vi "NI_controller_Feedback.VI"(1 "Initialize":bool=TRUE, 6 "Z Position (mm)":dbl format="%.3f", 8 "Motion System":T1=enum."No Motion Card", 9 "Y Position (mm)":dbl format="%.3f", 10 "X Position (mm)":dbl format="%.3f", 11 "Motion ID":T2=1 min=1 max=32 step=1) -> (0 "error out":errorcluster)   [LabVIEW 2022 SP3]
uses:
  <vilib>/Motion/FlexMotion/CustomControls/CustomControls.llb/AxisOrVectorSpace To Configure.flx
  <vilib>/Motion/FlexMotion/FunctionsVIs/StartStopMotion.llb/Start Motion (8 axes).flx
  <vilib>/Motion/FlexMotion/FunctionsVIs/StartStopMotion.llb/Stop Motion (8 axes).flx
  -MotionRoutines/MotionGlobals.vi
  <vilib>/Motion/FlexMotion/FunctionsVIs/Trajectory.llb/Load Acceleration/Deceleration.flx
  -NI_MotionRoutines/MotionSys.ctl
panel:
  in  "Slave Axis":u16(ring)=2 items=["Axis 1"=1, "Axis 2"=2, "Axis 3"=3, "Axis 4"=4]
  in  "Master Axis":u16(ring)=1 items=["Axis 1"=1, "Axis 2"=2, "Axis 3"=3, "Axis 4"=4]
  in  "Enable Gearing":bool
  out "Angle":dbl=45.000038009906035
  in  "Ratio Denom":u16=1 min=1 max=32767
  in  "Ratio Num":i16 min=0
  in  "Center 4":bool
  in  "Acceleration":i32=100000
  in  "Velocity":i32=20000
  in  "Position":dbl format="%.3f"
  in  "FineMi4":bool
  in  "FinePl4":bool
  in  "Rst4":bool
  in  "Ax4Plus":bool
  in  "Ax4Minus":bool
  in  "FineMi3":bool
  in  "FinePl3":bool
  in  "Rst3":bool
  in  "Ax3Plus":bool
  in  "Ax3Minus":bool
  in  "FineMi2":bool
  in  "FinePl2":bool
  in  "Rst2":bool
  in  "Ax2Plus":bool
  in  "Ax2Minus":bool
  in  "stop":bool
  in  "FineMi1":bool
  in  "FinePl1":bool
  in  "Rst1":bool
  in  "Ax1Plus":bool
  in  "Ax1Minus":bool
  # "Units are in mm. \"Rst\" zeros the position. Blue circles move 1 cm for linear."
  # "Be very careful with this mode it is not fully programmed"
  # "X Axis"
  # "Y Axis"
  # "Centers linear actuator"
  # "Z Axis"
  # "LinInd/Rotational Axis"
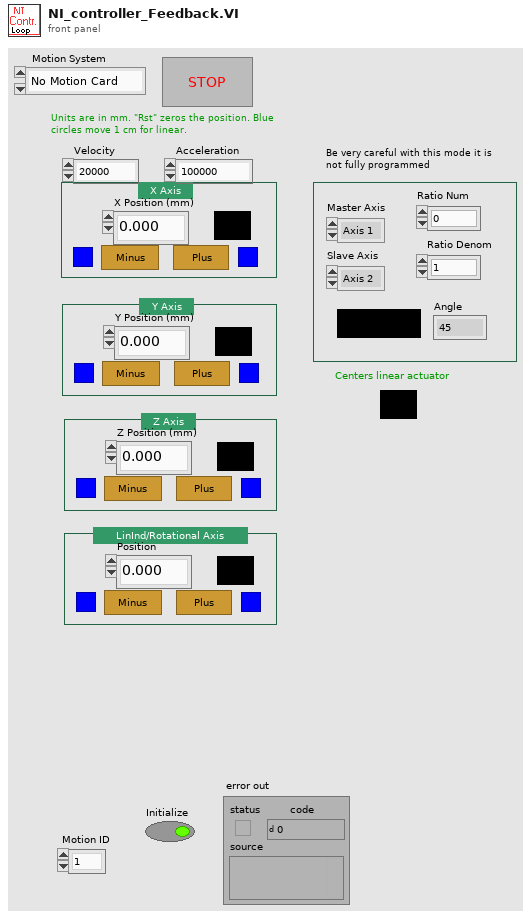
[diagram p1: front panel]
types:
  T1 = typedef "MotionSys.ctl" = enum16{"MM3000", "NI 735x", "Newport ESP", "No Motion Card", "Galil"}
  T2 = typedef "Board Id" = u8
  T3 = typedef "Bd Id Out" = u8
  T4 = typedef "location.ctl" = enum16{"Automatic", "WCM Main", "Hawaii", "Columbia MM3000", "Columbia  NI System", "NYU", "RRI 2", "UHI Allen", "CUMC RT", "Chiba", "Stony Brook", "WCM Microscopy", "WCM Aeoretch", "WCM Optics Lab", "WCM Main 2Axis", "WCM Rotation", "WCM SAM SMAC", "SERI GP"}
  T5 = typedef "AxisOrVectorSpace To Configure.flx" = u16
  T6 = enum16{"Absolute Position", "Relative Position", "Velocity", "Relative to Cap Pos", "Modulus Position", "Absolute Contouring", "Relative Contouring"}
  T7 = typedef "Resource Out (Enum).flx" = u16
  T8 = typedef "Axis Status (8 axes).flx" = cluster{"1":bool, "2":bool, "3":bool, "4":bool, "5":bool, "6":bool, "7":bool, "8":bool}
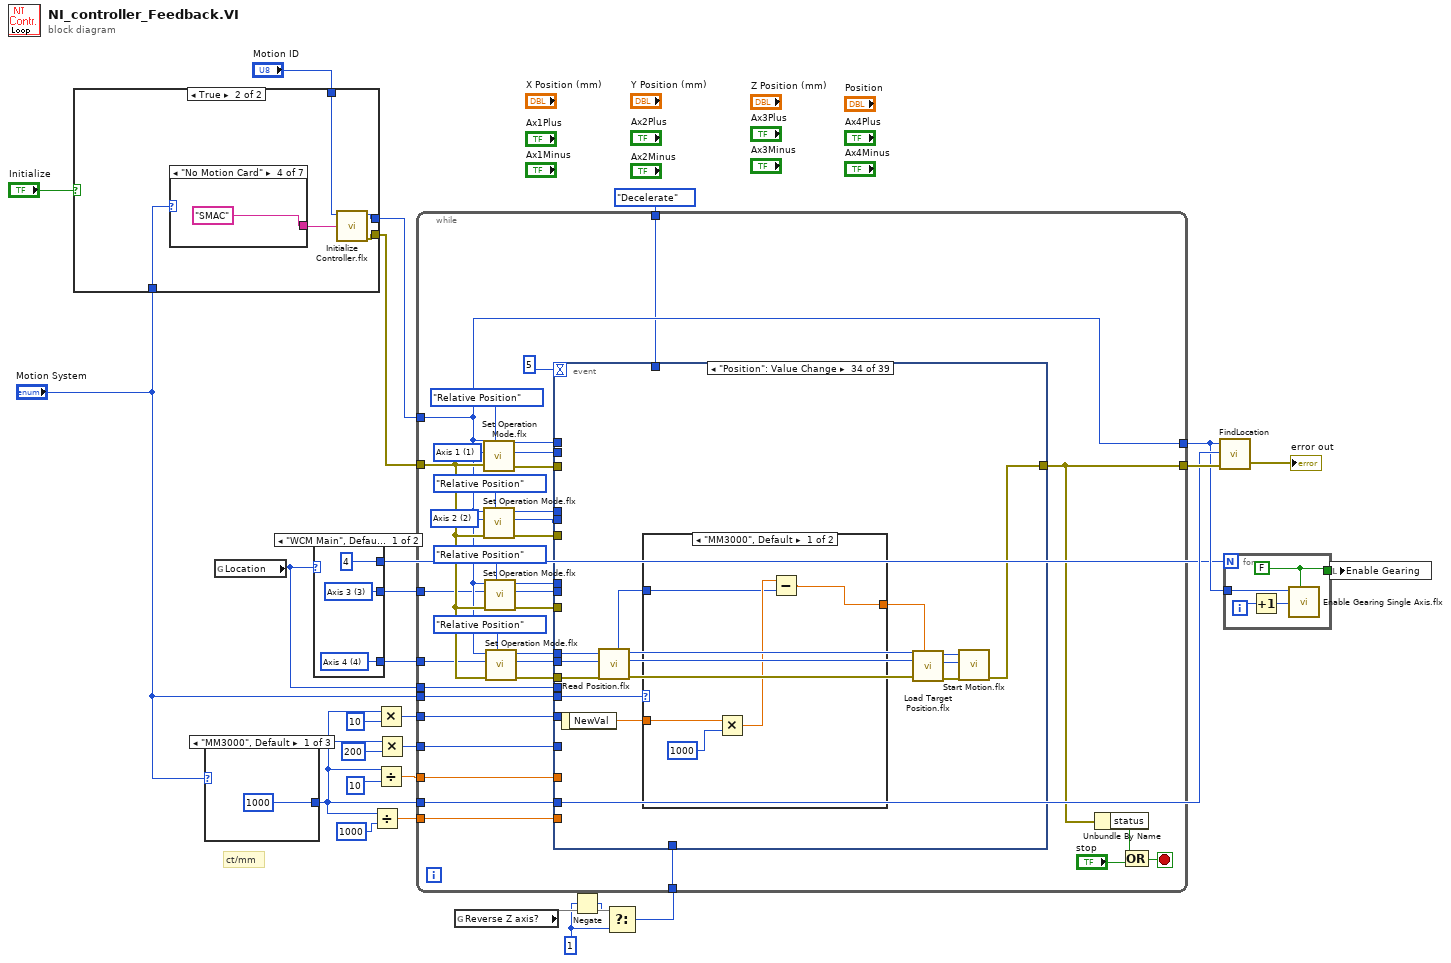
[diagram p0: block diagram]
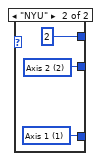
[diagram p2: hidden frame]
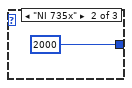
[diagram p3: hidden frame]
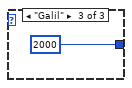
[diagram p4: hidden frame]
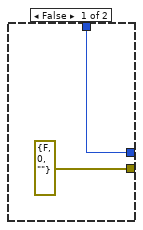
[diagram p5: hidden frame]
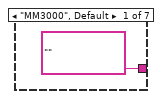
[diagram p6: hidden frame]
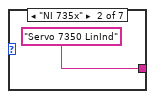
[diagram p7: hidden frame]
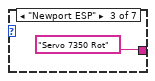
[diagram p8: hidden frame]
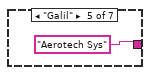
[diagram p9: hidden frame]
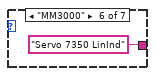
[diagram p10: hidden frame]
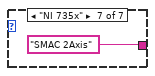
[diagram p11: hidden frame]
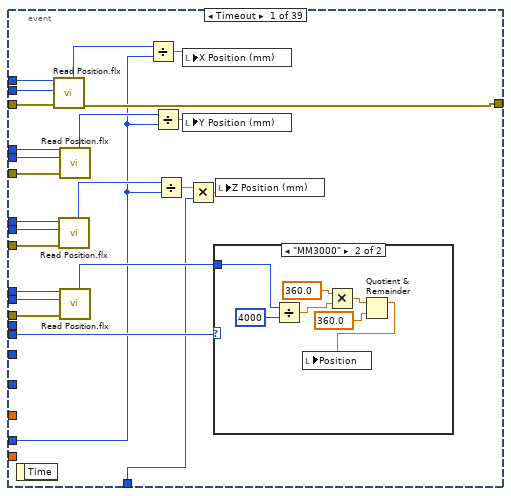
[diagram p12: hidden frame]
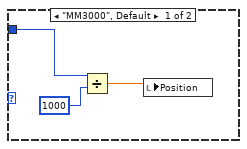
[diagram p13: hidden frame]
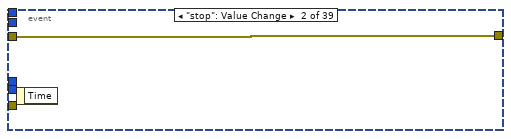
[diagram p14: hidden frame]
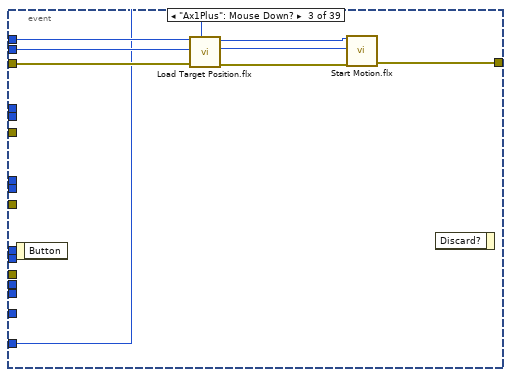
[diagram p15: hidden frame]
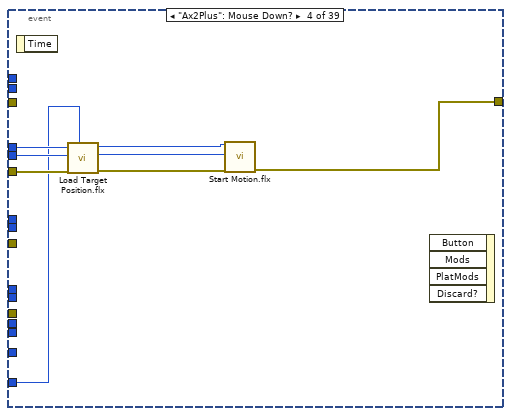
[diagram p16: hidden frame]
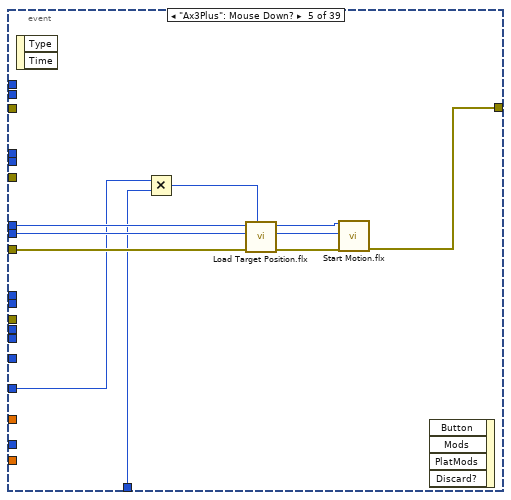
[diagram p17: hidden frame]
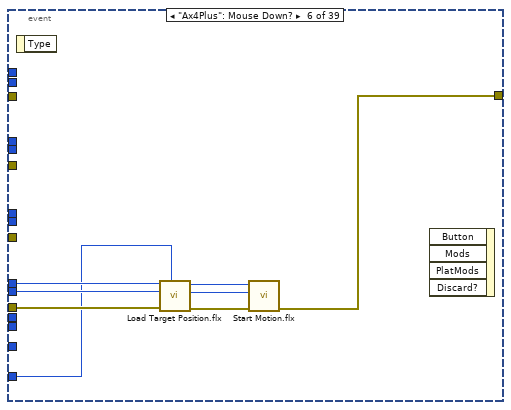
[diagram p18: hidden frame]
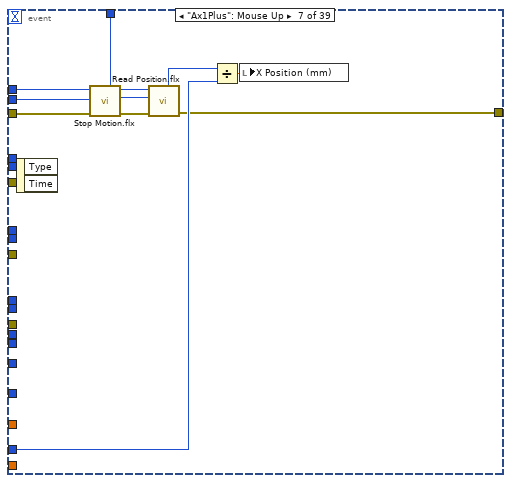
[diagram p19: hidden frame]
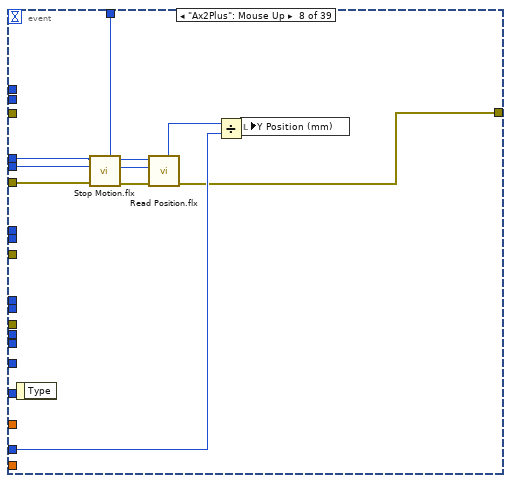
[diagram p20: hidden frame]
diagram:
  w12 = 1
  # "ct/mm"
  n1 = case shown="True" "Initialize" {
    tunnel: [w29 w34] -> w27
    tunnel: [errorcluster {"status"=FALSE, "code"=0, "source"=""} ("error out") w33] -> w26
    tunnel: "Motion ID" -> [w29 w31]
    tunnel: "Motion System" -> [_ w30]
    frame False {
    }
    frame True {
      n2 = case shown="\"No Motion Card\"" w30 {
        tunnel: ["" "Servo 7350 LinInd" "Servo 7350 Rot" "SMAC" "Aerotech Sys" "Servo 7350 LinInd" "SMAC 2Axis"] -> w32
        frame "MM3000", Default {
        }
        frame "NI 735x" {
        }
        frame "Newport ESP" {
        }
        frame "No Motion Card" {
        }
        frame "Galil" {
        }
        frame "MM3000" {
        }
        frame "NI 735x" {
        }
      }
      n3 = call <vilib>:"Initialize Controller.flx"("Settings Name"=w32, "Board ID"=w31) -> ("error out"=w33:errorcluster, "Bd ID Out"=w34:T3)  [unwired: 1 in, 5 out]
    }
  }
  n4 = case shown="\"MM3000\", Default" "Motion System" {
    tunnel: [1000 ("y") 2000 ("y") 2000 ("y")] -> w7
    frame "MM3000", Default {
    }
    frame "NI 735x" {
    }
    frame "Galil" {
    }
  }
  n5 = global read "MotionGlobals.vi" "Location"() -> (w1:T4)
  n6 = case shown="\"WCM Main\", Default" w1 {
    tunnel: [w47 w49] -> w4
    tunnel: [w46 w50] -> w3
    tunnel: [4 2] -> w2
    frame "WCM Main", Default {
      w47 = T5 4 items=["Axis 1"=1, "Axis 2"=2, "Axis 3"=3, "Axis 4"=4, "Axis 5"=5, "Axis 6"=6, "Vector Space 1"=17, "Vector Space 2"=18, "Vector Space 3"=19] ("Axis or Vector Space")
      w46 = T5 3 items=["Axis 1"=1, "Axis 2"=2, "Axis 3"=3, "Axis 4"=4, "Axis 5"=5, "Axis 6"=6, "Vector Space 1"=17, "Vector Space 2"=18, "Vector Space 3"=19] ("Axis or Vector Space")
    }
    frame "NYU" {
      w49 = T5 1 items=["Axis 1"=1, "Axis 2"=2, "Axis 3"=3, "Axis 4"=4, "Axis 5"=5, "Axis 6"=6, "Vector Space 1"=17, "Vector Space 2"=18, "Vector Space 3"=19] ("Axis or Vector Space")
      w50 = T5 2 items=["Axis 1"=1, "Axis 2"=2, "Axis 3"=3, "Axis 4"=4, "Axis 5"=5, "Axis 6"=6, "Vector Space 1"=17, "Vector Space 2"=18, "Vector Space 3"=19] ("Axis or Vector Space")
    }
  }
  n7 = Divide(x=w7, y=1000) -> (x/y=w10:dbl)
  n8 = Multiply(x=w7, y=10) -> (x*y=w14:i32)
  n9 = Divide(x=w7, y=10) -> (x/y=w17:dbl)
  n10 = Multiply(x=w7, y=200) -> (x*y=w13:i32)
  n11 = global read "MotionGlobals.vi" "Reverse Z axis?"() -> (w22)
  n12 = Negate(x=w12) -> (-x=w21:i32)
  n13 = Select(t=w21, s=w22, f=w12) -> (s? t:f=w20:i32)
  n14 = while {
    tunnel: [w58] -> w23
    tunnel: w26 -> [w74]
    tunnel: w27 -> [w66]
    tunnel: [w66] -> w6
    tunnel: w20 -> [w62]
    tunnel: w17 -> [w61]
    tunnel: w7 -> [w60]
    tunnel: "Motion System" -> [w59]
    tunnel: w14 -> [w57]
    tunnel: w13 -> [w56]
    tunnel: w10 -> [w55]
    tunnel: enum16{"Decelerate", "Halt", "Kill"}."Decelerate" ("Stop Type (Decel)") -> [w54]
    tunnel: w4 -> [w53]
    tunnel: w3 -> [w52]
    tunnel: w1 -> [w51]
    stop <- w85 stop-if-true
    w63 = T5 2 items=["Axis 1"=1, "Axis 2"=2, "Axis 3"=3, "Axis 4"=4, "Axis 5"=5, "Axis 6"=6, "Vector Space 1"=17, "Vector Space 2"=18, "Vector Space 3"=19] ("Axis or Vector Space")
    w79 = T5 1 items=["Axis 1"=1, "Axis 2"=2, "Axis 3"=3, "Axis 4"=4, "Axis 5"=5, "Axis 6"=6, "Vector Space 1"=17, "Vector Space 2"=18, "Vector Space 3"=19] ("Axis or Vector Space")
    n15 = call <vilib>:"Set Operation Mode.flx"("Position Mode (Absolute)"=T6."Relative Position", "error in (no error)"=w74, "Axis or Vector Space"=w79, "Board ID"=w66) -> ("error out"=w81:errorcluster, "Resource Output"=w78:T7, "Bd ID Out"=w82:T3)  [unwired: 2 out]
    n16 = call <vilib>:"Set Operation Mode.flx"("Position Mode (Absolute)"=T6."Relative Position", "error in (no error)"=w74, "Axis or Vector Space"=w63, "Board ID"=w66) -> ("error out"=w73:errorcluster, "Resource Output"=w65:T7, "Bd ID Out"=w64:T3)  [unwired: 2 out]
    n17 = call <vilib>:"Set Operation Mode.flx"("Position Mode (Absolute)"=T6."Relative Position", "error in (no error)"=w74, "Axis or Vector Space"=w52, "Board ID"=w66) -> ("error out"=w70:errorcluster, "Resource Output"=w71:T7, "Bd ID Out"=w72:T3)  [unwired: 2 out]
    n18 = call <vilib>:"Set Operation Mode.flx"("Position Mode (Absolute)"=T6."Relative Position", "error in (no error)"=w74, "Axis or Vector Space"=w53, "Board ID"=w66) -> ("error out"=w67:errorcluster, "Resource Output"=w68:T7, "Bd ID Out"=w69:T3)  [unwired: 2 out]
    n19 = event shown="[33] \"Position\": Value Change" {
      selector: _ -> [_ _ _ _ _ _ _ _ _ _ _ _ _ _ _ _ _ _ _ _ _ _ _ _ _ _ _ _ _ _ _ _ _ _ _ _ _ _ _]
      dyn-events: _ -> [_ _ _ _ _ _ _ _ _ _ _ _ _ _ _ _ _ _ _ _ _ _ _ _ _ _ _ _ _ _ _ _ _ _ _ _ _ _ _]
      timeout: 5 -> [_ _ _ _ _ _ _ _ _ _ _ _ _ _ _ _ _ _ _ _ _ _ _ _ _ _ _ _ _ _ _ _ _ _ _ _ _ _ _]
      tunnel: w82 -> [w110 _ w129 _ _ _ w166 _ _ _ w227 _ _ _ w266 _ _ _ w324 _ _ _ w344 _ _ _ w400 _ _ _ w468 _ _ _ _ _ _ _ _]
      tunnel: w81 -> [w108 w121 w127 _ _ _ w165 _ _ _ w225 _ _ _ w265 _ _ _ w323 _ _ _ w342 _ _ _ w398 _ _ _ w466 _ _ _ _ _ _ _ _]
      tunnel: w54 -> [_ _ _ _ _ _ w164 w173 w186 w200 _ _ _ _ w267 w274 w287 w298 _ _ _ _ _ _ _ _ _ _ _ _ _ _ _ _ _ _ _ _ _]
      tunnel: w78 -> [w109 _ w128 _ _ _ w158 _ _ _ w226 _ _ _ w259 _ _ _ w322 _ _ _ w343 _ _ _ w399 _ _ _ w467 _ _ _ _ _ _ _ _]
      tunnel: w64 -> [w104 _ _ w134 _ _ _ w172 _ _ _ w233 _ _ _ w273 _ _ _ w329 _ _ _ w352 _ _ _ w409 _ _ _ w474 _ _ _ _ _ w655 w665]
      tunnel: w65 -> [w94 _ _ w133 _ _ _ w171 _ _ _ w232 _ _ _ w272 _ _ _ w328 _ _ _ w351 _ _ _ w408 _ _ _ w472 _ _ _ _ _ _ _]
      tunnel: w73 -> [w103 _ _ w132 _ _ _ w170 _ _ _ w231 _ _ _ w271 _ _ _ w327 _ _ _ w350 _ _ _ w407 _ _ _ w473 _ _ _ _ _ _ _]
      tunnel: w72 -> [w102 _ _ _ w144 _ _ _ w185 _ _ _ w244 _ _ _ w286 _ _ _ w334 _ _ _ w362 _ _ _ w420 _ _ _ w491 _ _ _ _ _ _]
      tunnel: w71 -> [w101 _ _ _ w143 _ _ _ w184 _ _ _ w243 _ _ _ w285 _ _ _ w333 _ _ _ w361 _ _ _ w419 _ _ _ w490 _ _ _ _ _ _]
      tunnel: w70 -> [w100 _ _ _ w142 _ _ _ w183 _ _ _ w242 _ _ _ w284 _ _ _ w332 _ _ _ w360 _ _ _ w418 _ _ _ w489 _ _ _ _ _ _]
      tunnel: w69 -> [w99 _ _ _ _ w152 _ _ _ w199 _ _ _ w253 _ _ _ w297 _ _ _ w339 _ _ _ w370 _ _ _ w428 _ _ _ w508 w541 w579 w622 _ _]
      tunnel: w68 -> [w98 _ _ _ _ w151 _ _ _ w198 _ _ _ w252 _ _ _ w296 _ _ _ w338 _ _ _ w369 _ _ _ w427 _ _ _ w507 w534 w572 w621 _ _]
      tunnel: w67 -> [w97 _ _ _ _ w150 _ _ _ w197 _ _ _ w251 _ _ _ w295 _ _ _ w337 _ _ _ w368 _ _ _ w426 _ _ _ w506 w543 w582 w620 _ _]
      tunnel: [w91 w121 w123 w131 w139 w149 w156 w167 w182 w191 w221 w230 w238 w250 w257 w268 w283 w292 w320 w325 w330 _ w341 w349 w357 w367 w397 w406 w415 w425 w454 w470 w487 w503 w538 w577 _ _ _] -> w58
      tunnel: [_ _ _ _ _ _ _ _ _ _ _ _ _ _ _ _ _ _ _ _ _ w336 _ _ _ _ _ _ _ _ _ _ _ _ _ _ _ _ _] -> _
      tunnel: w62 -> [w88 _ _ _ w141 _ _ _ w178 _ _ _ w241 _ _ _ w280 _ _ _ _ _ _ _ w359 _ _ _ w417 _ _ _ w486 _ _ _ _ _ _]
      tunnel: w61 -> [_ _ _ _ _ _ _ _ _ _ _ _ _ _ _ _ _ _ _ _ _ _ _ _ _ _ _ _ _ _ _ _ _ _ _ _ _ _ _]
      tunnel: w60 -> [w87 _ _ _ _ _ w157 w168 w180 _ _ _ _ _ w258 w269 w279 _ _ _ _ _ _ _ _ _ _ _ _ _ w453 w469 w485 _ _ _ _ _ _]
      tunnel: w59 -> [w92 _ _ _ _ _ _ _ _ w192 _ _ _ _ _ _ _ w293 _ _ _ _ _ _ _ w366 _ _ _ w424 _ _ _ w502 w536 w574 _ _ _]
      tunnel: w57 -> [_ _ _ _ _ _ _ _ _ _ _ _ _ _ _ _ _ _ _ _ _ _ w340 w348 w356 _ w396 w405 w414 _ _ _ _ _ _ _ _ _ _]
      tunnel: w56 -> [_ _ w122 w130 w138 w148 _ _ _ _ w220 w229 w237 w249 _ _ _ _ _ _ _ _ _ _ _ _ _ _ _ _ _ _ _ _ _ _ _ _ _]
      tunnel: w55 -> [_ _ _ _ _ _ _ _ _ _ _ _ _ _ _ _ _ _ _ _ _ _ _ _ _ _ _ _ _ _ _ _ _ _ w542 w580 _ _ _]
      tunnel: w51 -> [_ _ _ _ _ _ _ _ _ _ _ _ _ _ _ _ _ _ _ _ _ _ _ _ _ _ _ _ _ _ _ _ _ _ w533 w571 w609 _ _]
      event Timeout {
        n20 = event-data() -> ()  [unwired: 2 out]
        n21 = call <vilib>:"Read Position.flx"("error in (no error)"=w108, "Axis"=w109, "Board ID"=w110) -> ("error out"=w91:errorcluster, "Position"=w107:i32)  [unwired: 5 out]
        n22 = call <vilib>:"Read Position.flx"("error in (no error)"=w100, "Axis"=w101, "Board ID"=w102) -> ("Position"=w90:i32)  [unwired: 6 out]
        n23 = call <vilib>:"Read Position.flx"("error in (no error)"=w103, "Axis"=w94, "Board ID"=w104) -> ("Position"=w105:i32)  [unwired: 6 out]
        n24 = call <vilib>:"Read Position.flx"("error in (no error)"=w97, "Axis"=w98, "Board ID"=w99) -> ("Position"=w93:i32)  [unwired: 6 out]
        n25 = Divide(x=w107, y=w87) -> (x/y=w106:dbl)
        n26 = Divide(x=w105, y=w87) -> (x/y=w96:dbl)
        n27 = Divide(x=w90, y=w87) -> (x/y=w89:dbl)
        n28 = local write "X Position (mm)"(w106) -> ()
        n29 = local write "Y Position (mm)"(w96) -> ()
        n30 = Multiply(x=w89, y=w88) -> (x*y=w95:dbl)
        n31 = case shown="\"50\"" w92 {
          tunnel: w93 -> [w113 w114]
          frame "MM3000", Default {
            n32 = Divide(x=w113, y=1000) -> (x/y=w111:dbl)
            n33 = local write "Position"(w111) -> ()
          }
          frame "MM3000" {
            n34 = Divide(x=w114, y=4000) -> (x/y=w119:dbl)
            n35 = Multiply(x=360.0, y=w119) -> (x*y=w116:dbl)
            n36 = Quotient & Remainder(x=w116, y=360.0) -> (x-y*floor(x/y)=w115:dbl)  [unwired: 1 out]
            n37 = local write "Position"(w115) -> ()
          }
        }
        n38 = local write "Z Position (mm)"(w95) -> ()
      }
      event "stop": Value Change {
        n39 = event-data() -> ()  [unwired: 2 out]
      }
      event "Ax1Plus": Mouse Down? {
        n40 = event-data() -> ()  [unwired: 2 out]
        n41 = call <vilib>:"Load Target Position.flx"("Target Position (0)"=w122, "error in (no error)"=w127, "Axis"=w128, "Board ID"=w129) -> ("error out"=w126:errorcluster, "Resource Output"=w125:T7, "Bd ID Out"=w124:T3)  [unwired: 3 out]
        n42 = call-poly <vilib>:"Start Motion.flx"("error in (no error)"=w126, "Axis or Vector Space"=w125, "Board ID"=w124) -> ("error out"=w123:errorcluster)  [unwired: 1 in, 4 out]
        n43 = event-data() -> ()  [unwired: 1 in, 2 out]
      }
      event "Ax2Plus": Mouse Down? {
        n44 = event-data() -> ()  [unwired: 2 out]
        n45 = call <vilib>:"Load Target Position.flx"("Target Position (0)"=w130, "error in (no error)"=w132, "Axis"=w133, "Board ID"=w134) -> ("error out"=w137:errorcluster, "Resource Output"=w136:T7, "Bd ID Out"=w135:T3)  [unwired: 3 out]
        n46 = call-poly <vilib>:"Start Motion.flx"("error in (no error)"=w137, "Axis or Vector Space"=w136, "Board ID"=w135) -> ("error out"=w131:errorcluster)  [unwired: 1 in, 4 out]
        n47 = event-data() -> ()  [unwired: 1 in, 5 out]
      }
      event "Ax3Plus": Mouse Down? {
        n48 = event-data() -> ()  [unwired: 3 out]
        n49 = Multiply(x=w138, y=w141) -> (x*y=w140:i32)
        n50 = call <vilib>:"Load Target Position.flx"("Target Position (0)"=w140, "error in (no error)"=w142, "Axis"=w143, "Board ID"=w144) -> ("error out"=w147:errorcluster, "Resource Output"=w146:T7, "Bd ID Out"=w145:T3)  [unwired: 3 out]
        n51 = call-poly <vilib>:"Start Motion.flx"("error in (no error)"=w147, "Axis or Vector Space"=w146, "Board ID"=w145) -> ("error out"=w139:errorcluster)  [unwired: 1 in, 4 out]
        n52 = event-data() -> ()  [unwired: 1 in, 5 out]
      }
      event "Ax4Plus": Mouse Down? {
        n53 = event-data() -> ()  [unwired: 2 out]
        n54 = call <vilib>:"Load Target Position.flx"("Target Position (0)"=w148, "error in (no error)"=w150, "Axis"=w151, "Board ID"=w152) -> ("error out"=w155:errorcluster, "Resource Output"=w154:T7, "Bd ID Out"=w153:T3)  [unwired: 3 out]
        n55 = call-poly <vilib>:"Start Motion.flx"("error in (no error)"=w155, "Axis or Vector Space"=w154, "Board ID"=w153) -> ("error out"=w149:errorcluster)  [unwired: 1 in, 4 out]
        n56 = event-data() -> ()  [unwired: 1 in, 5 out]
      }
      event "Ax1Plus": Mouse Up {
        n57 = event-data() -> ()  [unwired: 3 out]
        n58 = call-poly <vilib>:"Stop Motion.flx"("Stop Type (Decel)"=w164, "error in (no error)"=w165, "Axis or Vector Space"=w158, "Board ID"=w166) -> ("error out"=w161:errorcluster, "Resource Output"=w162:T7, "Bd ID Out"=w163:T3)  [unwired: 1 in, 2 out]
        n59 = call <vilib>:"Read Position.flx"("error in (no error)"=w161, "Axis"=w162, "Board ID"=w163) -> ("error out"=w156:errorcluster, "Position"=w160:i32)  [unwired: 5 out]
        n60 = Divide(x=w160, y=w157) -> (x/y=w159:dbl)
        n61 = local write "X Position (mm)"(w159) -> ()
      }
      event "Ax2Plus": Mouse Up {
        n62 = event-data() -> ()  [unwired: 2 out]
        n63 = call-poly <vilib>:"Stop Motion.flx"("Stop Type (Decel)"=w173, "error in (no error)"=w170, "Axis or Vector Space"=w171, "Board ID"=w172) -> ("error out"=w175:errorcluster, "Resource Output"=w176:T7, "Bd ID Out"=w177:T3)  [unwired: 1 in, 2 out]
        n64 = call <vilib>:"Read Position.flx"("error in (no error)"=w175, "Axis"=w176, "Board ID"=w177) -> ("error out"=w167:errorcluster, "Position"=w174:i32)  [unwired: 5 out]
        n65 = Divide(x=w174, y=w168) -> (x/y=w169:dbl)
        n66 = local write "Y Position (mm)"(w169) -> ()
      }
      event "Ax3Plus": Mouse Up {
        n67 = event-data() -> ()  [unwired: 2 out]
        n68 = call-poly <vilib>:"Stop Motion.flx"("Stop Type (Decel)"=w186, "error in (no error)"=w183, "Axis or Vector Space"=w184, "Board ID"=w185) -> ("error out"=w189:errorcluster, "Resource Output"=w188:T7, "Bd ID Out"=w187:T3)  [unwired: 1 in, 2 out]
        n69 = call <vilib>:"Read Position.flx"("error in (no error)"=w189, "Axis"=w188, "Board ID"=w187) -> ("error out"=w182:errorcluster, "Position"=w190:i32)  [unwired: 5 out]
        n70 = Divide(x=w190, y=w180) -> (x/y=w181:dbl)
        n71 = Multiply(x=w181, y=w178) -> (x*y=w179:dbl)
        n72 = local write "Z Position (mm)"(w179) -> ()
      }
      event "Ax4Plus": Mouse Up {
        n73 = event-data() -> ()  [unwired: 2 out]
        n74 = call-poly <vilib>:"Stop Motion.flx"("Stop Type (Decel)"=w200, "error in (no error)"=w197, "Axis or Vector Space"=w198, "Board ID"=w199) -> ("error out"=w194:errorcluster, "Resource Output"=w195:T7, "Bd ID Out"=w196:T3)  [unwired: 1 in, 2 out]
        n75 = case shown="\"MM3000\", Default" w192 {
          tunnel: w196 -> [w205 w211]
          tunnel: w195 -> [w204 w210]
          tunnel: w194 -> [w203 w212]
          tunnel: [w202 w209] -> w191
          tunnel: [w201 w208] -> w193
          frame "MM3000", Default {
            n76 = call <vilib>:"Read Position.flx"("error in (no error)"=w203, "Axis"=w204, "Board ID"=w205) -> ("error out"=w202:errorcluster, "Position"=w206:i32)  [unwired: 5 out]
            n77 = Divide(x=w206, y=1000) -> (x/y=w201:dbl)
          }
          frame "MM3000" {
            n78 = call <vilib>:"Read Position.flx"("error in (no error)"=w212, "Axis"=w210, "Board ID"=w211) -> ("error out"=w209:errorcluster, "Position"=w214:i32)  [unwired: 5 out]
            n79 = Divide(x=w214, y=4000) -> (x/y=w215:dbl)
            n80 = Multiply(x=360.0, y=w215) -> (x*y=w217:dbl)
            n81 = Quotient & Remainder(x=w217, y=360.0) -> (x-y*floor(x/y)=w208:dbl)  [unwired: 1 out]
          }
        }
        n82 = local write "Position"(w193) -> ()
      }
      event "Ax1Minus": Mouse Down? {
        n83 = event-data() -> ()  [unwired: 2 out]
        n84 = Negate(x=w220) -> (-x=w219:i32)
        n85 = call <vilib>:"Load Target Position.flx"("Target Position (0)"=w219, "error in (no error)"=w225, "Axis"=w226, "Board ID"=w227) -> ("error out"=w224:errorcluster, "Resource Output"=w223:T7, "Bd ID Out"=w222:T3)  [unwired: 3 out]
        n86 = call-poly <vilib>:"Start Motion.flx"("error in (no error)"=w224, "Axis or Vector Space"=w223, "Board ID"=w222) -> ("error out"=w221:errorcluster)  [unwired: 1 in, 4 out]
        n87 = event-data() -> ()  [unwired: 1 in, 2 out]
      }
      event "Ax2Minus": Mouse Down? {
        n88 = event-data() -> ()  [unwired: 2 out]
        n89 = Negate(x=w229) -> (-x=w228:i32)
        n90 = call <vilib>:"Load Target Position.flx"("Target Position (0)"=w228, "error in (no error)"=w231, "Axis"=w232, "Board ID"=w233) -> ("error out"=w236:errorcluster, "Resource Output"=w235:T7, "Bd ID Out"=w234:T3)  [unwired: 3 out]
        n91 = call-poly <vilib>:"Start Motion.flx"("error in (no error)"=w236, "Axis or Vector Space"=w235, "Board ID"=w234) -> ("error out"=w230:errorcluster)  [unwired: 1 in, 4 out]
        n92 = event-data() -> ()  [unwired: 1 in, 5 out]
      }
      event "Ax3Minus": Mouse Down? {
        n93 = event-data() -> ()  [unwired: 2 out]
        n94 = Negate(x=w237) -> (-x=w239:i32)
        n95 = Multiply(x=w239, y=w241) -> (x*y=w240:i32)
        n96 = call <vilib>:"Load Target Position.flx"("Target Position (0)"=w240, "error in (no error)"=w242, "Axis"=w243, "Board ID"=w244) -> ("error out"=w247:errorcluster, "Resource Output"=w246:T7, "Bd ID Out"=w245:T3)  [unwired: 3 out]
        n97 = call-poly <vilib>:"Start Motion.flx"("error in (no error)"=w247, "Axis or Vector Space"=w246, "Board ID"=w245) -> ("error out"=w238:errorcluster)  [unwired: 1 in, 4 out]
        n98 = event-data() -> ()  [unwired: 1 in, 5 out]
      }
      event "Ax4Minus": Mouse Down? {
        n99 = event-data() -> ()  [unwired: 2 out]
        n100 = Negate(x=w249) -> (-x=w248:i32)
        n101 = call <vilib>:"Load Target Position.flx"("Target Position (0)"=w248, "error in (no error)"=w251, "Axis"=w252, "Board ID"=w253) -> ("error out"=w254:errorcluster, "Resource Output"=w255:T7, "Bd ID Out"=w256:T3)  [unwired: 3 out]
        n102 = call-poly <vilib>:"Start Motion.flx"("error in (no error)"=w254, "Axis or Vector Space"=w255, "Board ID"=w256) -> ("error out"=w250:errorcluster)  [unwired: 1 in, 4 out]
        n103 = event-data() -> ()  [unwired: 1 in, 5 out]
      }
      event "Ax1Minus": Mouse Up {
        n104 = event-data() -> ()  [unwired: 4 out]
        n105 = call-poly <vilib>:"Stop Motion.flx"("Stop Type (Decel)"=w267, "error in (no error)"=w265, "Axis or Vector Space"=w259, "Board ID"=w266) -> ("error out"=w262:errorcluster, "Resource Output"=w263:T7, "Bd ID Out"=w264:T3)  [unwired: 1 in, 2 out]
        n106 = call <vilib>:"Read Position.flx"("error in (no error)"=w262, "Axis"=w263, "Board ID"=w264) -> ("error out"=w257:errorcluster, "Position"=w261:i32)  [unwired: 5 out]
        n107 = Divide(x=w261, y=w258) -> (x/y=w260:dbl)
        n108 = local write "X Position (mm)"(w260) -> ()
      }
      event "Ax2Minus": Mouse Up {
        n109 = event-data() -> ()  [unwired: 8 out]
        n110 = call-poly <vilib>:"Stop Motion.flx"("Stop Type (Decel)"=w274, "error in (no error)"=w271, "Axis or Vector Space"=w272, "Board ID"=w273) -> ("error out"=w277:errorcluster, "Resource Output"=w276:T7, "Bd ID Out"=w275:T3)  [unwired: 1 in, 2 out]
        n111 = call <vilib>:"Read Position.flx"("error in (no error)"=w277, "Axis"=w276, "Board ID"=w275) -> ("error out"=w268:errorcluster, "Position"=w278:i32)  [unwired: 5 out]
        n112 = Divide(x=w278, y=w269) -> (x/y=w270:dbl)
        n113 = local write "Y Position (mm)"(w270) -> ()
      }
      event "Ax3Minus": Mouse Up {
        n114 = event-data() -> ()  [unwired: 2 out]
        n115 = call-poly <vilib>:"Stop Motion.flx"("Stop Type (Decel)"=w287, "error in (no error)"=w284, "Axis or Vector Space"=w285, "Board ID"=w286) -> ("error out"=w290:errorcluster, "Resource Output"=w289:T7, "Bd ID Out"=w288:T3)  [unwired: 1 in, 2 out]
        n116 = call <vilib>:"Read Position.flx"("error in (no error)"=w290, "Axis"=w289, "Board ID"=w288) -> ("error out"=w283:errorcluster, "Position"=w291:i32)  [unwired: 5 out]
        n117 = Divide(x=w291, y=w279) -> (x/y=w282:dbl)
        n118 = Multiply(x=w282, y=w280) -> (x*y=w281:dbl)
        n119 = local write "Z Position (mm)"(w281) -> ()
      }
      event "Ax4Minus": Mouse Up {
        n120 = event-data() -> ()  [unwired: 2 out]
        n121 = call-poly <vilib>:"Stop Motion.flx"("Stop Type (Decel)"=w298, "error in (no error)"=w295, "Axis or Vector Space"=w296, "Board ID"=w297) -> ("error out"=w299:errorcluster, "Resource Output"=w300:T7, "Bd ID Out"=w301:T3)  [unwired: 1 in, 2 out]
        n122 = case shown="\"50\"" w293 {
          tunnel: w301 -> [w312 w317]
          tunnel: w300 -> [w311 w316]
          tunnel: w299 -> [w310 w315]
          tunnel: [w305 w314] -> w292
          tunnel: [w302 w313] -> w294
          frame "MM3000" {
            n123 = call <vilib>:"Read Position.flx"("error in (no error)"=w310, "Axis"=w311, "Board ID"=w312) -> ("error out"=w305:errorcluster, "Position"=w308:i32)  [unwired: 5 out]
            n124 = Divide(x=w308, y=4000) -> (x/y=w307:dbl)
            n125 = Multiply(x=360.0, y=w307) -> (x*y=w303:dbl)
            n126 = Quotient & Remainder(x=w303, y=360.0) -> (x-y*floor(x/y)=w302:dbl)  [unwired: 1 out]
          }
          frame "MM3000", Default {
            n127 = call <vilib>:"Read Position.flx"("error in (no error)"=w315, "Axis"=w316, "Board ID"=w317) -> ("error out"=w314:errorcluster, "Position"=w319:i32)  [unwired: 5 out]
            n128 = Divide(x=w319, y=1000) -> (x/y=w313:dbl)
          }
        }
        n129 = local write "Position"(w294) -> ()
      }
      event "Rst1": Value Change {
        w321 = 0 ("Primary Reset Position (0)")
        n130 = event-data() -> ()  [unwired: 3 out]
        n131 = call <vilib>:"Reset Position.flx"("Primary Reset Position (0)"=w321, "error in (no error)"=w323, "Axis"=w322, "Board ID"=w324) -> ("error out"=w320:errorcluster)  [unwired: 1 in, 4 out]
        n132 = local write "X Position (mm)"(w321) -> ()
      }
      event "Rst2": Value Change {
        w326 = 0 ("Primary Reset Position (0)")
        n133 = event-data() -> ()  [unwired: 4 out]
        n134 = call <vilib>:"Reset Position.flx"("Primary Reset Position (0)"=w326, "error in (no error)"=w327, "Axis"=w328, "Board ID"=w329) -> ("error out"=w325:errorcluster)  [unwired: 1 in, 4 out]
        n135 = local write "Y Position (mm)"(w326) -> ()
      }
      event "Rst3": Value Change {
        w331 = 0 ("Primary Reset Position (0)")
        n136 = event-data() -> ()  [unwired: 4 out]
        n137 = call <vilib>:"Reset Position.flx"("Primary Reset Position (0)"=w331, "error in (no error)"=w332, "Axis"=w333, "Board ID"=w334) -> ("error out"=w330:errorcluster)  [unwired: 1 in, 4 out]
        n138 = local write "Z Position (mm)"(w331) -> ()
      }
      event "Rst4": Value Change {
        w335 = 0 ("Primary Reset Position (0)")
        n139 = event-data() -> ()  [unwired: 6 out]
        n140 = call <vilib>:"Reset Position.flx"("Primary Reset Position (0)"=w335, "error in (no error)"=w337, "Axis"=w338, "Board ID"=w339) -> ("error out"=w336:errorcluster)  [unwired: 1 in, 4 out]
        n141 = local write "Position"(w335) -> ()
      }
      event "FinePl1": Value Change {
        # "# of counts for 1cm"
        n142 = event-data() -> ()  [unwired: 2 out]
        n143 = call <vilib>:"Load Target Position.flx"("Target Position (0)"=w340, "error in (no error)"=w342, "Axis"=w343, "Board ID"=w344) -> ("error out"=w346:errorcluster, "Resource Output"=w345:T7, "Bd ID Out"=w347:T3)  [unwired: 3 out]
        n144 = call-poly <vilib>:"Start Motion.flx"("error in (no error)"=w346, "Axis or Vector Space"=w345, "Board ID"=w347) -> ("error out"=w341:errorcluster)  [unwired: 1 in, 4 out]
      }
      event "FinePl2": Value Change {
        # "# of counts for 1cm"
        n145 = event-data() -> ()  [unwired: 2 out]
        n146 = call <vilib>:"Load Target Position.flx"("Target Position (0)"=w348, "error in (no error)"=w350, "Axis"=w351, "Board ID"=w352) -> ("error out"=w354:errorcluster, "Resource Output"=w353:T7, "Bd ID Out"=w355:T3)  [unwired: 3 out]
        n147 = call-poly <vilib>:"Start Motion.flx"("error in (no error)"=w354, "Axis or Vector Space"=w353, "Board ID"=w355) -> ("error out"=w349:errorcluster)  [unwired: 1 in, 4 out]
      }
      event "FinePl3": Value Change {
        # "# of counts for 1cm"
        n148 = event-data() -> ()  [unwired: 2 out]
        n149 = Multiply(x=w356, y=w359) -> (x*y=w358:i32)
        n150 = call <vilib>:"Load Target Position.flx"("Target Position (0)"=w358, "error in (no error)"=w360, "Axis"=w361, "Board ID"=w362) -> ("error out"=w364:errorcluster, "Resource Output"=w363:T7, "Bd ID Out"=w365:T3)  [unwired: 3 out]
        n151 = call-poly <vilib>:"Start Motion.flx"("error in (no error)"=w364, "Axis or Vector Space"=w363, "Board ID"=w365) -> ("error out"=w357:errorcluster)  [unwired: 1 in, 4 out]
      }
      event "FinePl4": Value Change {
        n152 = event-data() -> ()  [unwired: 6 out]
        n153 = case shown="\"Galil\"" w366 {
          tunnel: w370 -> [w374 w382 w390]
          tunnel: w369 -> [w373 w381 w389]
          tunnel: w368 -> [w372 w380 w388]
          tunnel: [w371 w379 w387] -> w367
          frame "MM3000", Default {
            # "# of counts for 1cm"
            n154 = call <vilib>:"Load Target Position.flx"("Target Position (0)"=10000 ("x"), "error in (no error)"=w372, "Axis"=w373, "Board ID"=w374) -> ("error out"=w377:errorcluster, "Resource Output"=w376:T7, "Bd ID Out"=w378:T3)  [unwired: 3 out]
            n155 = call-poly <vilib>:"Start Motion.flx"("error in (no error)"=w377, "Axis or Vector Space"=w376, "Board ID"=w378) -> ("error out"=w371:errorcluster)  [unwired: 1 in, 4 out]
          }
          frame "Newport ESP" {
            # "# of counts for 1 revolution"
            n156 = call <vilib>:"Load Target Position.flx"("Target Position (0)"=4000 ("x"), "error in (no error)"=w380, "Axis"=w381, "Board ID"=w382) -> ("error out"=w385:errorcluster, "Resource Output"=w384:T7, "Bd ID Out"=w386:T3)  [unwired: 3 out]
            n157 = call-poly <vilib>:"Start Motion.flx"("error in (no error)"=w385, "Axis or Vector Space"=w384, "Board ID"=w386) -> ("error out"=w379:errorcluster)  [unwired: 1 in, 4 out]
          }
          frame "Galil" {
            # "# of counts for 1 revolution"
            n158 = call <vilib>:"Load Target Position.flx"("Target Position (0)"=4000 ("x"), "error in (no error)"=w388, "Axis"=w389, "Board ID"=w390) -> ("error out"=w393:errorcluster, "Resource Output"=w392:T7, "Bd ID Out"=w394:T3)  [unwired: 3 out]
            n159 = call-poly <vilib>:"Start Motion.flx"("error in (no error)"=w393, "Axis or Vector Space"=w392, "Board ID"=w394) -> ("error out"=w387:errorcluster)  [unwired: 1 in, 4 out]
          }
        }
      }
      event "FineMi1": Value Change {
        # "# of counts for 1cm"
        n160 = event-data() -> ()  [unwired: 4 out]
        n161 = Negate(x=w396) -> (-x=w395:i32)
        n162 = call <vilib>:"Load Target Position.flx"("Target Position (0)"=w395, "error in (no error)"=w398, "Axis"=w399, "Board ID"=w400) -> ("error out"=w402:errorcluster, "Resource Output"=w403:T7, "Bd ID Out"=w401:T3)  [unwired: 3 out]
        n163 = call-poly <vilib>:"Start Motion.flx"("error in (no error)"=w402, "Axis or Vector Space"=w403, "Board ID"=w401) -> ("error out"=w397:errorcluster)  [unwired: 1 in, 4 out]
      }
      event "FineMi2": Value Change {
        # "# of counts for 1cm"
        n164 = event-data() -> ()  [unwired: 4 out]
        n165 = Negate(x=w405) -> (-x=w404:i32)
        n166 = call <vilib>:"Load Target Position.flx"("Target Position (0)"=w404, "error in (no error)"=w407, "Axis"=w408, "Board ID"=w409) -> ("error out"=w411:errorcluster, "Resource Output"=w412:T7, "Bd ID Out"=w410:T3)  [unwired: 3 out]
        n167 = call-poly <vilib>:"Start Motion.flx"("error in (no error)"=w411, "Axis or Vector Space"=w412, "Board ID"=w410) -> ("error out"=w406:errorcluster)  [unwired: 1 in, 4 out]
      }
      event "FineMi3": Value Change {
        # "# of counts for 1cm"
        n168 = event-data() -> ()  [unwired: 4 out]
        n169 = Negate(x=w414) -> (-x=w413:i32)
        n170 = Multiply(x=w413, y=w417) -> (x*y=w416:i32)
        n171 = call <vilib>:"Load Target Position.flx"("Target Position (0)"=w416, "error in (no error)"=w418, "Axis"=w419, "Board ID"=w420) -> ("error out"=w422:errorcluster, "Resource Output"=w423:T7, "Bd ID Out"=w421:T3)  [unwired: 3 out]
        n172 = call-poly <vilib>:"Start Motion.flx"("error in (no error)"=w422, "Axis or Vector Space"=w423, "Board ID"=w421) -> ("error out"=w415:errorcluster)  [unwired: 1 in, 4 out]
      }
      event "FineMi4": Value Change {
        n173 = event-data() -> ()  [unwired: 6 out]
        n174 = case shown="\"Galil\"" w424 {
          tunnel: w428 -> [w432 w440 w448]
          tunnel: w427 -> [w431 w439 w447]
          tunnel: w426 -> [w430 w438 w446]
          tunnel: [w429 w437 w445] -> w425
          frame "MM3000", Default {
            # "# of counts for 1cm"
            n175 = call <vilib>:"Load Target Position.flx"("Target Position (0)"=-10000 ("x"), "error in (no error)"=w430, "Axis"=w431, "Board ID"=w432) -> ("error out"=w434:errorcluster, "Resource Output"=w435:T7, "Bd ID Out"=w433:T3)  [unwired: 3 out]
            n176 = call-poly <vilib>:"Start Motion.flx"("error in (no error)"=w434, "Axis or Vector Space"=w435, "Board ID"=w433) -> ("error out"=w429:errorcluster)  [unwired: 1 in, 4 out]
          }
          frame "Newport ESP" {
            # "# of counts for 1 revolution"
            n177 = call <vilib>:"Load Target Position.flx"("Target Position (0)"=-4000 ("x"), "error in (no error)"=w438, "Axis"=w439, "Board ID"=w440) -> ("error out"=w442:errorcluster, "Resource Output"=w443:T7, "Bd ID Out"=w441:T3)  [unwired: 3 out]
            n178 = call-poly <vilib>:"Start Motion.flx"("error in (no error)"=w442, "Axis or Vector Space"=w443, "Board ID"=w441) -> ("error out"=w437:errorcluster)  [unwired: 1 in, 4 out]
          }
          frame "Galil" {
            # "# of counts for 1 revolution"
            n179 = call <vilib>:"Load Target Position.flx"("Target Position (0)"=-4000 ("x"), "error in (no error)"=w446, "Axis"=w447, "Board ID"=w448) -> ("error out"=w450:errorcluster, "Resource Output"=w451:T7, "Bd ID Out"=w449:T3)  [unwired: 3 out]
            n180 = call-poly <vilib>:"Start Motion.flx"("error in (no error)"=w450, "Axis or Vector Space"=w451, "Board ID"=w449) -> ("error out"=w445:errorcluster)  [unwired: 1 in, 4 out]
          }
        }
      }
      event "X Position (mm)": Value Change {
        n181 = event-data() -> ("NewVal"=w455:dbl)  [unwired: 1 out]
        n182 = call <vilib>:"Read Position.flx"("error in (no error)"=w466, "Axis"=w467, "Board ID"=w468) -> ("error out"=w463:errorcluster, "Resource Output"=w464:T7, "Bd ID Out"=w465:T3, "Position"=w462:i32)  [unwired: 3 out]
        n183 = Multiply(x=w455, y=w453) -> (x*y=w461:dbl)
        n184 = Subtract(x=w461, y=w462) -> (x-y=w460:dbl)
        n185 = To Long Integer(number=w460) -> (32bit integer=w459:i32)
        n186 = call <vilib>:"Load Target Position.flx"("Target Position (0)"=w459, "error in (no error)"=w463, "Axis"=w464, "Board ID"=w465) -> ("error out"=w456:errorcluster, "Resource Output"=w457:T7, "Bd ID Out"=w458:T3)  [unwired: 3 out]
        n187 = call-poly <vilib>:"Start Motion.flx"("error in (no error)"=w456, "Axis or Vector Space"=w457, "Board ID"=w458) -> ("error out"=w454:errorcluster)  [unwired: 1 in, 4 out]
      }
      event "Y Position (mm)": Value Change {
        n188 = event-data() -> ("NewVal"=w471:dbl)  [unwired: 1 out]
        n189 = call <vilib>:"Read Position.flx"("error in (no error)"=w473, "Axis"=w472, "Board ID"=w474) -> ("error out"=w482:errorcluster, "Resource Output"=w483:T7, "Bd ID Out"=w484:T3, "Position"=w481:i32)  [unwired: 3 out]
        n190 = Multiply(x=w471, y=w469) -> (x*y=w480:dbl)
        n191 = Subtract(x=w480, y=w481) -> (x-y=w479:dbl)
        n192 = To Long Integer(number=w479) -> (32bit integer=w478:i32)
        n193 = call <vilib>:"Load Target Position.flx"("Target Position (0)"=w478, "error in (no error)"=w482, "Axis"=w483, "Board ID"=w484) -> ("error out"=w475:errorcluster, "Resource Output"=w476:T7, "Bd ID Out"=w477:T3)  [unwired: 3 out]
        n194 = call-poly <vilib>:"Start Motion.flx"("error in (no error)"=w475, "Axis or Vector Space"=w476, "Board ID"=w477) -> ("error out"=w470:errorcluster)  [unwired: 1 in, 4 out]
      }
      event "Z Position (mm)": Value Change {
        n195 = event-data() -> ("NewVal"=w488:dbl)  [unwired: 1 out]
        n196 = call <vilib>:"Read Position.flx"("error in (no error)"=w489, "Axis"=w490, "Board ID"=w491) -> ("error out"=w499:errorcluster, "Resource Output"=w500:T7, "Bd ID Out"=w501:T3, "Position"=w498:i32)  [unwired: 3 out]
        n197 = Compound Arithmetic op=MULTIPLY(w488, w485, w486) -> (w497:dbl)
        n198 = Subtract(x=w497, y=w498) -> (x-y=w496:dbl)
        n199 = To Long Integer(number=w496) -> (32bit integer=w495:i32)
        n200 = call <vilib>:"Load Target Position.flx"("Target Position (0)"=w495, "error in (no error)"=w499, "Axis"=w500, "Board ID"=w501) -> ("error out"=w492:errorcluster, "Resource Output"=w493:T7, "Bd ID Out"=w494:T3)  [unwired: 3 out]
        n201 = call-poly <vilib>:"Start Motion.flx"("error in (no error)"=w492, "Axis or Vector Space"=w493, "Board ID"=w494) -> ("error out"=w487:errorcluster)  [unwired: 1 in, 4 out]
      }
      event "Position": Value Change {
        n202 = event-data() -> ("NewVal"=w504:dbl)  [unwired: 1 out]
        n203 = call <vilib>:"Read Position.flx"("error in (no error)"=w506, "Axis"=w507, "Board ID"=w508) -> ("error out"=w513:errorcluster, "Resource Output"=w514:T7, "Bd ID Out"=w515:T3, "Position"=w505:i32)  [unwired: 3 out]
        n204 = case shown="\"MM3000\", Default" w502 {
          tunnel: [w517 w523] -> w512
          tunnel: w505 -> [w518 w529]
          tunnel: w504 -> [w519 w524]
          frame "MM3000", Default {
            n205 = Multiply(x=w519, y=1000) -> (x*y=w520:dbl)
            n206 = Subtract(x=w520, y=w518) -> (x-y=w517:dbl)
          }
          frame "MM3000" {
            w522 = 360.0 ("y")
            w521 = 4000 ("y")
            n207 = Divide(x=w529, y=w521) -> (x/y=w528:dbl)
            n208 = Multiply(x=w528, y=w522) -> (x*y=w527:dbl)
            n209 = Quotient & Remainder(x=w524, y=w522) -> (x-y*floor(x/y)=w530:dbl)  [unwired: 1 out]
            n210 = Divide(x=w530, y=w522) -> (x/y=w531:dbl)
            n211 = Quotient & Remainder(x=w527, y=w522) -> (x-y*floor(x/y)=w526:dbl)  [unwired: 1 out]
            n212 = Multiply(x=w526, y=w521) -> (x*y=w525:dbl)
            n213 = Multiply(x=w531, y=w521) -> (x*y=w532:dbl)
            n214 = Subtract(x=w532, y=w525) -> (x-y=w523:dbl)
          }
        }
        n215 = call <vilib>:"Load Target Position.flx"("Target Position (0)"=w512, "error in (no error)"=w513, "Axis"=w514, "Board ID"=w515) -> ("error out"=w509:errorcluster, "Resource Output"=w510:T7, "Bd ID Out"=w511:T3)  [unwired: 3 out]
        n216 = call-poly <vilib>:"Start Motion.flx"("error in (no error)"=w509, "Axis or Vector Space"=w510, "Board ID"=w511) -> ("error out"=w503:errorcluster)  [unwired: 1 in, 4 out]
      }
      event "Velocity": Value Change {
        n217 = event-data() -> ()  [unwired: 2 out]
        n218 = Multiply(x="Velocity", y=w542) -> (x*y=w540:dbl)
        n219 = case shown="\"NYU\"" w533 {
          tunnel: w543 -> [w549 w563]
          tunnel: w541 -> [w548 w562]
          tunnel: w540 -> [w547 w561]
          tunnel: [w546 w560] -> w539
          tunnel: [w545 w559] -> w537
          frame "WCM Main", Default {
            n220 = for {
              N: 3 -> [_]
              tunnel: w549 -> [w555]
              tunnel: [w554] -> w546
              tunnel: w547 -> [w552]
              tunnel: w548 -> [w553]
              tunnel: [w551] -> w545
              i -> [w557]
              n221 = Increment(x=w557) -> (x+1=w556:i32)
              n222 = call <vilib>:"Load Velocity.flx"("Velocity (10000)"=w552, "error in (no error)"=w555, "Axis or Vector Space"=w556, "Board ID"=w553) -> ("error out"=w554:errorcluster, "Bd ID Out"=w551:T3)  [unwired: 4 out]
            }
          }
          frame "NYU" {
            w558 = T5 2 items=["Axis 1"=1, "Axis 2"=2, "Axis 3"=3, "Axis 4"=4, "Axis 5"=5, "Axis 6"=6, "Vector Space 1"=17, "Vector Space 2"=18, "Vector Space 3"=19] ("Axis or Vector Space")
            n223 = call <vilib>:"Load Velocity.flx"("Velocity (10000)"=w561, "error in (no error)"=w563, "Axis or Vector Space"=w558, "Board ID"=w562) -> ("error out"=w560:errorcluster, "Bd ID Out"=w559:T3)  [unwired: 4 out]
          }
        }
        n224 = global write "MotionGlobals.vi" "motor velocity"(w540) -> ()
        n225 = case shown="\"Newport ESP\"" w536 {
          tunnel: w540 -> [w564 w566 w569]
          tunnel: [w564 w565 w568] -> _
          frame "MM3000", Default {
          }
          frame "Newport ESP" {
            n226 = Divide(x=w566, y=20) -> (x/y=w565:dbl)
          }
          frame "Galil" {
            n227 = Divide(x=w569, y=20) -> (x/y=w568:dbl)
          }
        }
        n228 = call <vilib>:"Load Velocity.flx"("Velocity (10000)"=40000, "error in (no error)"=w539, "Axis or Vector Space"=w534, "Board ID"=w537) -> ("error out"=w538:errorcluster)  [unwired: 5 out]
      }
      event "Acceleration": Value Change {
        n229 = event-data() -> ()  [unwired: 2 out]
        n230 = Multiply(x="Acceleration", y=w580) -> (x*y=w573:dbl)
        n231 = case shown="\"WCM Main\", Default" w571 {
          tunnel: w582 -> [w587 w601]
          tunnel: w579 -> [w586 w600]
          tunnel: [w585 w599] -> w578
          tunnel: [w584 w598] -> w576
          tunnel: w573 -> [w583 w597]
          frame "WCM Main", Default {
            n232 = for {
              N: 3 -> [_]
              tunnel: w587 -> [w593]
              tunnel: [w592] -> w585
              tunnel: w583 -> [w590]
              tunnel: w586 -> [w591]
              tunnel: [w589] -> w584
              i -> [w595]
              n233 = Increment(x=w595) -> (x+1=w594:i32)
              n234 = call "Load Acceleration/Deceleration.flx"("Acceleration (100000)"=w590, "error in (no error)"=w593, "Axis or Vector Space"=w594, "Board ID"=w591) -> ("error out"=w592:errorcluster, "Bd ID Out"=w589:T3)  [unwired: 1 in, 3 out]
            }
          }
          frame "NYU" {
            w596 = T5 2 items=["Axis 1"=1, "Axis 2"=2, "Axis 3"=3, "Axis 4"=4, "Axis 5"=5, "Axis 6"=6, "Vector Space 1"=17, "Vector Space 2"=18, "Vector Space 3"=19] ("Axis or Vector Space")
            n235 = call "Load Acceleration/Deceleration.flx"("Acceleration (100000)"=w597, "error in (no error)"=w601, "Axis or Vector Space"=w596, "Board ID"=w600) -> ("error out"=w599:errorcluster, "Bd ID Out"=w598:T3)  [unwired: 1 in, 3 out]
          }
        }
        n236 = global write "MotionGlobals.vi" "motor accel"(w573) -> ()
        n237 = case shown="\"MM3000\", Default" w574 {
          tunnel: w573 -> [w602 w604 w607]
          tunnel: [w602 w603 w606] -> w575
          frame "MM3000", Default {
          }
          frame "Newport ESP" {
            n238 = Divide(x=w604, y=10) -> (x/y=w603:dbl)
          }
          frame "Galil" {
            n239 = Divide(x=w607, y=10) -> (x/y=w606:dbl)
          }
        }
        n240 = call "Load Acceleration/Deceleration.flx"("Acceleration (100000)"=w575, "error in (no error)"=w578, "Axis or Vector Space"=w572, "Board ID"=w576) -> ("error out"=w577:errorcluster)  [unwired: 1 in, 4 out]
      }
      event "Center 4": Value Change {
        w610 = T6."Relative Position" ("Position Mode (Absolute)")
        # "Center the motion stage"
        n241 = event-data() -> ()  [unwired: 7 out]
        n242 = call <vilib>:"Set Operation Mode.flx"("Position Mode (Absolute)"=w610, "error in (no error)"=w620, "Axis or Vector Space"=w621, "Board ID"=w622) -> ("error out"=w619:errorcluster, "Resource Output"=w617:T7, "Bd ID Out"=w618:T3)  [unwired: 2 out]
        n243 = call <vilib>:"Load Target Position.flx"("Target Position (0)"=24000, "error in (no error)"=w619, "Axis"=w617, "Board ID"=w618) -> ("error out"=w635:errorcluster, "Resource Output"=w634:T7, "Bd ID Out"=w633:T3)  [unwired: 3 out]
        n244 = call-poly <vilib>:"Start Motion.flx"("error in (no error)"=w635, "Axis or Vector Space"=w634, "Board ID"=w633) -> ("error out"=w630:errorcluster, "Resource Output"=w623:T7, "Bd ID Out"=w631:T3)  [unwired: 1 in, 2 out]
        n245 = while {
          tunnel: w631 -> [w645]
          tunnel: w630 -> [w644]
          tunnel: [w638] -> w628
          tunnel: [w637] -> w629
          tunnel: w609 -> [w636]
          stop <- w639 stop-if-true
          n246 = call <vilib>:"Read Limit Status.vi"("error in (no error)"=w644, "Board ID"=w645) -> ("error out"=w638:errorcluster, "Bd ID Out"=w637:T3, "Reverse Limits"=w643:T8, "Forward Limits"=w642:T8)  [unwired: 1 in, 5 out]
          n247 = case shown="\"NYU\"" w636 {
            tunnel: w643 -> [w649 w653]
            tunnel: w642 -> [w648 w652]
            tunnel: [w647 w651] -> w641
            tunnel: [w646 w650] -> w640
            frame "WCM Main", Default {
              n248 = Unbundle By Name(w649) -> ("4"=w647:bool)
              n249 = Unbundle By Name(w648) -> ("4"=w646:bool)
            }
            frame "NYU" {
              n250 = Unbundle By Name(w653) -> ("1"=w651:bool)
              n251 = Unbundle By Name(w652) -> ("1"=w650:bool)
            }
          }
          n252 = Or(x=w641, y=w640) -> (x .or. y?=w639:bool)
        }
        n253 = call-poly <vilib>:"Stop Motion.flx"("error in (no error)"=w628, "Axis or Vector Space"=w623, "Board ID"=w629) -> ("error out"=w615:errorcluster, "Resource Output"=w611:T7, "Bd ID Out"=w616:T3)  [unwired: 2 in, 2 out]
        n254 = call <vilib>:"Set Operation Mode.flx"("Position Mode (Absolute)"=w610, "error in (no error)"=w615, "Axis or Vector Space"=w611, "Board ID"=w616) -> ("error out"=w614:errorcluster, "Resource Output"=w612:T7, "Bd ID Out"=w613:T3)  [unwired: 2 out]
        n255 = call <vilib>:"Load Target Position.flx"("Target Position (0)"=-12000, "error in (no error)"=w614, "Axis"=w612, "Board ID"=w613) -> ("error out"=w627:errorcluster, "Resource Output"=w626:T7, "Bd ID Out"=w625:T3)  [unwired: 3 out]
        n256 = call-poly <vilib>:"Start Motion.flx"("error in (no error)"=w627, "Axis or Vector Space"=w626, "Board ID"=w625) -> ()  [unwired: 1 in, 5 out]
      }
      event "Ratio Num", "Ratio Denom", "Master Axis", "Slave Axis": Value Change {
        n257 = event-data() -> ()  [unwired: 7 out]
        n258 = call <vilib>:"Configure Gear Master.flx"("Master Axis Encoder or ADC"="Master Axis", "Axis"="Slave Axis", "Board ID"=w655) -> ("error out"=w661:errorcluster, "Resource Output"=w660:T7, "Bd ID Out"=w662:T3)  [unwired: 1 in, 2 out]
        n259 = call <vilib>:"Load Gear Ratio.flx"("Ratio Denominator (1)"="Ratio Denom", "Ratio Numerator (0)"="Ratio Num", "Gearing (Absolute)"=TRUE, "error in (no error)"=w661, "Axis"=w660, "Board ID"=w662) -> ()  [unwired: 6 out]
        n260 = Divide(x="Ratio Num", y="Ratio Denom") -> (x/y=w663:dbl)
        n261 = expression code="atan(x)*360/2/3.14159"(w663) -> (→"Angle":dbl)
      }
      event "Enable Gearing": Value Change {
        n262 = event-data() -> ()  [unwired: 7 out]
        n263 = local read "Slave Axis"() -> (w666:u16)
        n264 = call <vilib>:"Enable Gearing Single Axis.flx"("Gearing (Disable)"="Enable Gearing", "Axis"=w666, "Board ID"=w665) -> ()  [unwired: 1 in, 6 out]
      }
    }
    n265 = Unbundle By Name(w58) -> ("status"=w84:bool)
    n266 = Compound Arithmetic op=OR(w84, "stop") -> (w85:bool)
  }
  n267 = call "FindLocation.vi"("error in (no error)"=w23, "ct/mm"=w7, "Board ID"=w6) -> ("error out"=→"error out":errorcluster)  [unwired: 1 out]
  n268 = for {
    N: w2 -> [_]
    tunnel: w6 -> [w671]
    tunnel: [w668] -> w5
    i -> [w670]
    w668 = FALSE ("Gearing (Disable)")
    n269 = Increment(x=w670) -> (x+1=w669:i32)
    n270 = call <vilib>:"Enable Gearing Single Axis.flx"("Gearing (Disable)"=w668, "Axis"=w669, "Board ID"=w671) -> ()  [unwired: 1 in, 6 out]
  }
  n271 = local write "Enable Gearing"(w5) -> ()
